vi "GV DO4.vi"() -> ()   [LabVIEW 2017]
panel:
  out "DO4":bool
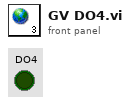
[diagram p1: front panel]
diagram:
